vi "Read Hostname.vi"(11 "Test Suite Result In":refnum<class "Test Suite Result.lvclass">) -> (2 "Hostname":string, 3 "Test Suite Result Out":refnum<class "Test Suite Result.lvclass">)   [LabVIEW 2020, in "Test Suite Result.lvclass"]
uses:
  Test Suite Result.lvclass
  Test Suite Result.lvclass/Test Suite Result.ctl
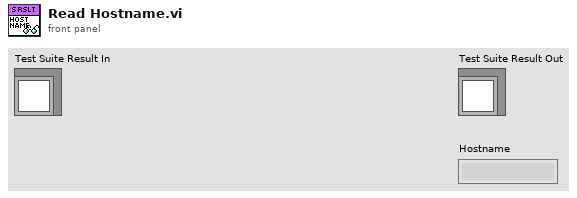
[diagram p1: front panel]
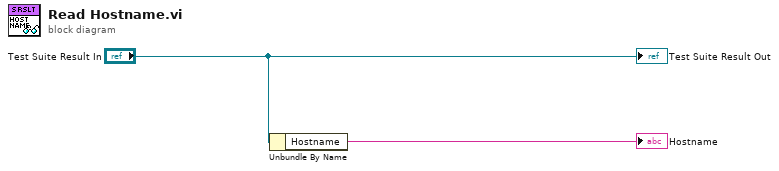
[diagram p0: block diagram]
diagram:
  n1 = Unbundle By Name("Test Suite Result In") -> ("Hostname"=→"Hostname":string)
  "Test Suite Result Out" <- "Test Suite Result In"
